vi "5492_PullContourNTValues.vi"(8 "Shapes Found":dbl, 11 "Max Value\nMax Value":string(combo)) -> (3 "Output Cluster":T1)   [LabVIEW 2016]
uses:
  <vilib>/Rock Robotics/Network Tables/NT Read Numeric Array.vi
panel:
  in  "Cluster":T1
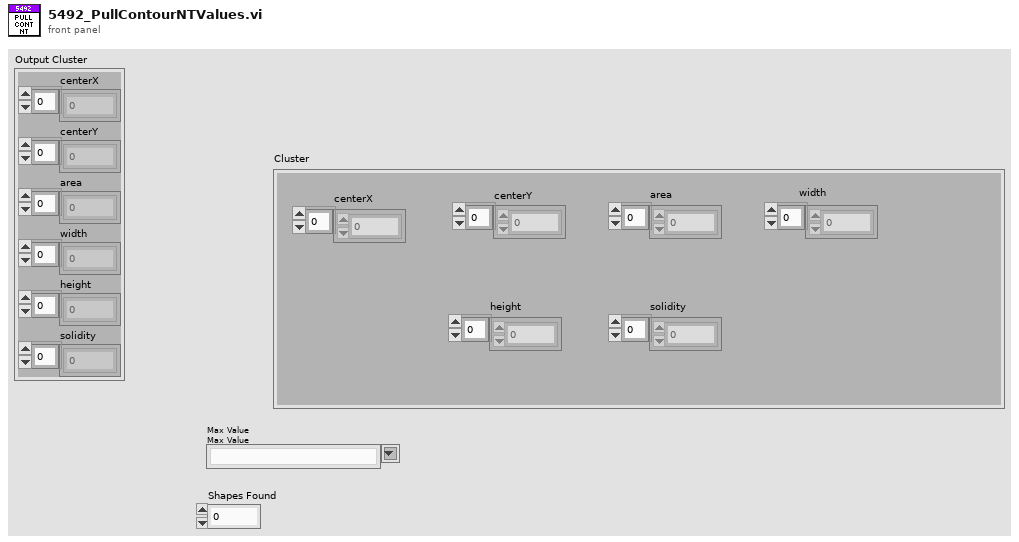
[diagram p1: front panel]
types:
  T1 = cluster{"centerX":dbl[], "centerY":dbl[], "area":dbl[], "width":dbl[], "height":dbl[], "solidity":dbl[]}
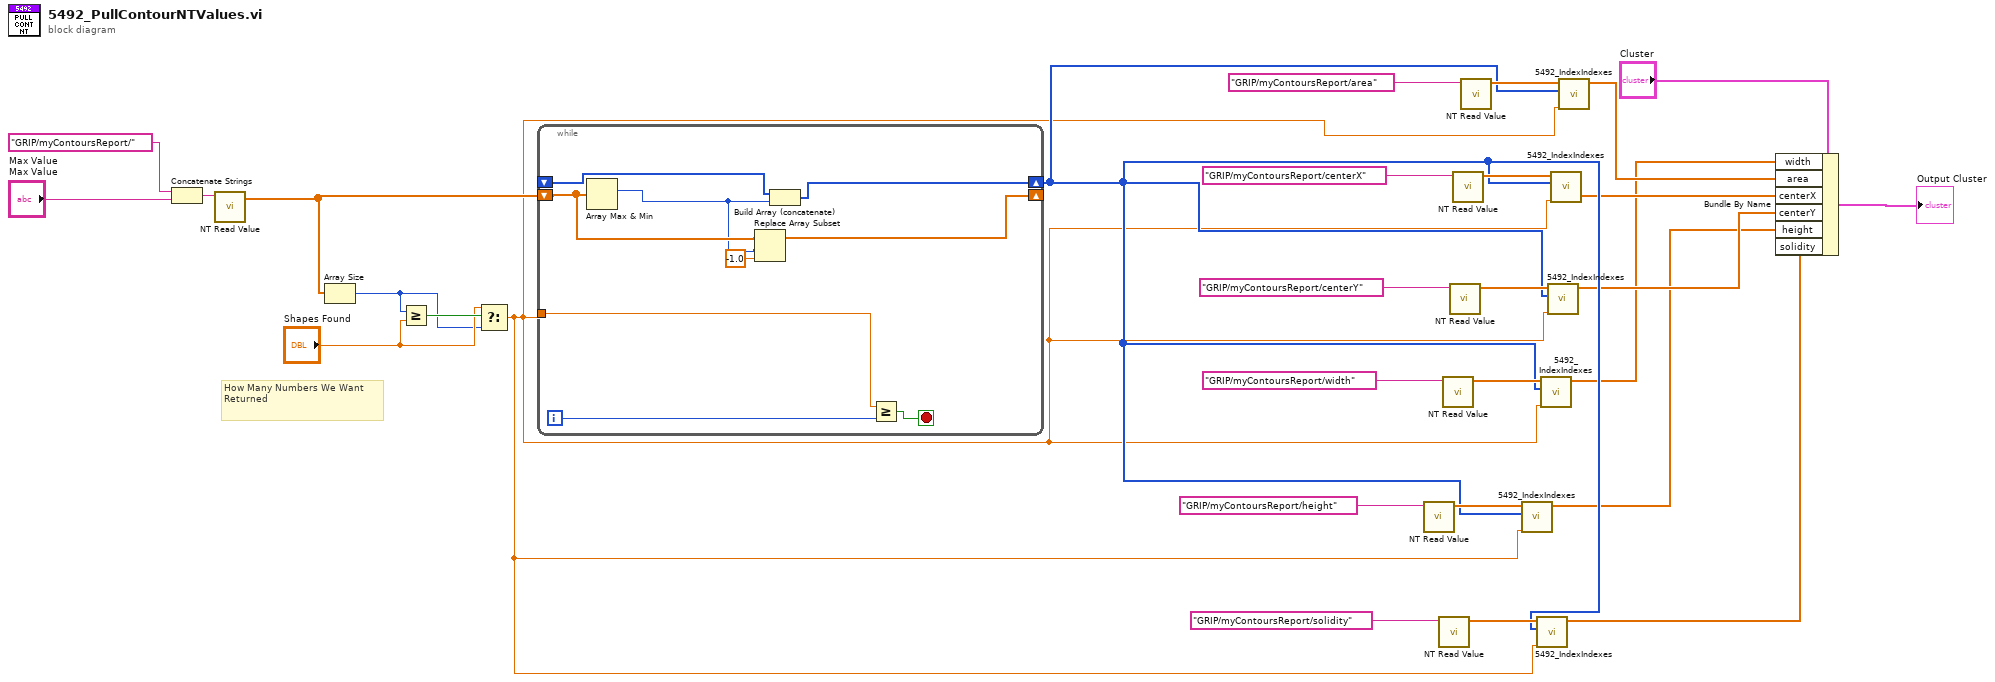
[diagram p0: block diagram]
diagram:
  # "How Many Numbers We Want \nReturned"
  n1 = Concatenate Strings("GRIP/myContoursReport/", "Max Value\nMax Value") -> (w27:string)
  n2 = call-poly <vilib>:"NT Read Value.vi"("Name"=w27) -> ("Numeric Array"=w23:dbl[])  [unwired: 9 in, 1 out]
  n3 = Array Size(array=w23) -> (size(s)=w24:i32)
  n4 = Greater Or Equal?(x=w24, y="Shapes Found") -> (x >= y?=w26:bool)
  n5 = Select(t="Shapes Found", s=w26, f=w24) -> (s? t:f=w9:dbl)
  n6 = while {
    shift-right: [w30] -> w10
    shift-left: _ -> [w38]
    tunnel: w9 -> [w36]
    shift-right: [w31] -> _
    shift-left: w23 -> [w35]
    i -> [w32]
    stop <- w37 stop-if-true
    n7 = Array Max & Min(array=w35) -> (max index (indices)=w34:i32)  [unwired: 3 out]
    n8 = Replace Array Subset(array=w35, new element=-1.0 ("new element/subarray"), index=w34) -> (w31:dbl[])
    n9 = Build Array (concatenate)(w38, w34) -> (w30:i32[])
    n10 = Greater Or Equal?(x=w36, y=w32) -> (x >= y?=w37:bool)
  }
  n11 = call-poly <vilib>:"NT Read Value.vi"("Name"="GRIP/myContoursReport/height") -> ("Numeric Array"=w12:dbl[])  [unwired: 9 in, 1 out]
  n12 = call-poly <vilib>:"NT Read Value.vi"("Name"="GRIP/myContoursReport/solidity") -> ("Numeric Array"=w11:dbl[])  [unwired: 9 in, 1 out]
  n13 = call-poly <vilib>:"NT Read Value.vi"("Name"="GRIP/myContoursReport/width") -> ("Numeric Array"=w13:dbl[])  [unwired: 9 in, 1 out]
  n14 = call-poly <vilib>:"NT Read Value.vi"("Name"="GRIP/myContoursReport/centerY") -> ("Numeric Array"=w14:dbl[])  [unwired: 9 in, 1 out]
  n15 = call-poly <vilib>:"NT Read Value.vi"("Name"="GRIP/myContoursReport/centerX") -> ("Numeric Array"=w16:dbl[])  [unwired: 9 in, 1 out]
  n16 = call-poly <vilib>:"NT Read Value.vi"("Name"="GRIP/myContoursReport/area") -> ("Numeric Array"=w15:dbl[])  [unwired: 9 in, 1 out]
  n17 = call "5492_IndexIndexes.vi"("Shapes Found"=w9, "Indexes"=w10, "Full Data"=w12) -> ("Output Array"=w5:dbl[])  [unwired: 8 in]
  n18 = call "5492_IndexIndexes.vi"("Shapes Found"=w9, "Indexes"=w10, "Full Data"=w11) -> ("Output Array"=w4:dbl[])  [unwired: 8 in]
  n19 = call "5492_IndexIndexes.vi"("Shapes Found"=w9, "Indexes"=w10, "Full Data"=w13) -> ("Output Array"=w3:dbl[])  [unwired: 8 in]
  n20 = call "5492_IndexIndexes.vi"("Shapes Found"=w9, "Indexes"=w10, "Full Data"=w14) -> ("Output Array"=w6:dbl[])  [unwired: 8 in]
  n21 = call "5492_IndexIndexes.vi"("Shapes Found"=w9, "Indexes"=w10, "Full Data"=w16) -> ("Output Array"=w7:dbl[])  [unwired: 8 in]
  n22 = call "5492_IndexIndexes.vi"("Shapes Found"=w9, "Indexes"=w10, "Full Data"=w15) -> ("Output Array"=w8:dbl[])  [unwired: 8 in]
  n23 = Bundle By Name(cluster="Cluster", "width"=w3, "area"=w8, "centerX"=w7, "centerY"=w6, "height"=w5, "solidity"=w4) -> (→"Output Cluster":T1)
